vi "公式节点.vi"() -> ()   [LabVIEW 2014]
panel:
  out "数值 3":dbl
  in  "下拉列表":u16(ring) items=["Apple"=1, "Banana"=2]
  out "数值 2":dbl
  in  "组合框":string(combo)
  out "数值":i16
  in  "b":i16(knob) scale=0.0..10.0
  in  "a":i16(knob) scale=0.0..10.0
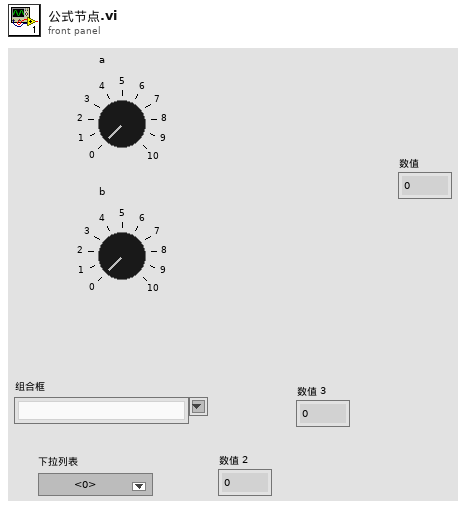
[diagram p1: front panel]
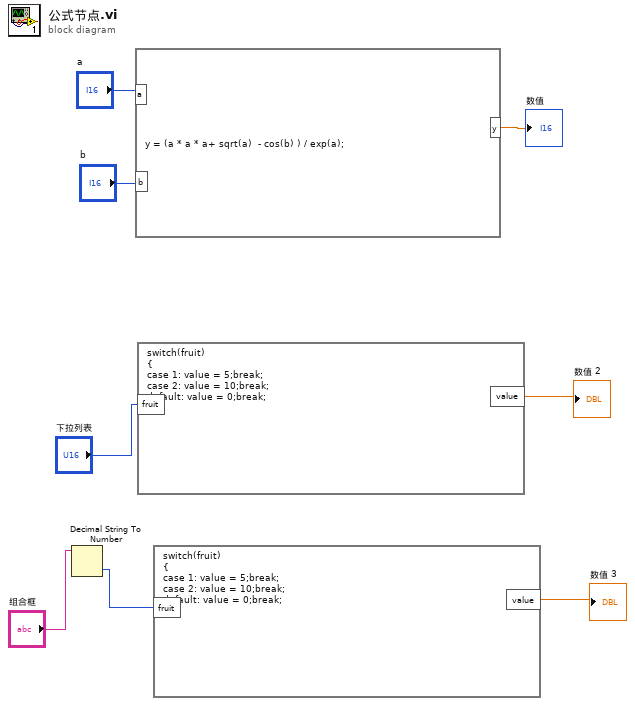
[diagram p0: block diagram]
diagram:
  n1 = Decimal String To Number(string="组合框") -> (number=w2:i32)  [unwired: 2 in, 1 out]
  n2 = formula code="y = (a * a * a+ sqrt(a)  - cos(b) ) / exp(a);"("a"="a", "b"="b") -> ("y"=→"数值":dbl)
  n3 = formula code="switch(fruit)\n{\ncase 1: value = 5;break;\ncase 2: value = 10;break;\ndefault: value = 0;break;\n}"("fruit"="下拉列表") -> ("value"=→"数值 2":dbl)
  n4 = formula code="switch(fruit)\n{\ncase 1: value = 5;break;\ncase 2: value = 10;break;\ndefault: value = 0;break;\n}"("fruit"=w2) -> ("value"=→"数值 3":dbl)
